vi "Write Target-FIFO 1ch.vi"(1 "FIFO In":refnum<k21>="FIFO-000", 5 "16IQ in":cluster{"I":fxp<+/-,18,1>, "Q":fxp<+/-,18,1>}[](array[cluster])=[{"I"=0.0, "Q"=0.0}, {"I"=0.0, "Q"=0.0}, {"I"=0.0, "Q"=0.0}, {"I"=0.0, "Q"=0.0}, {"I"=0.0, "Q"=0.0}, {"I"=0.0, "Q"=0.0}, {"I"=0.0, "Q"=0.0}, {"I"=0.0, "Q"=0.0}, {"I"=0.0, "Q"=0.0}, {"I"=0.0, "Q"=0.0}, {"I"=0.0, "Q"=0.0}, {"I"=0.0, "Q"=0.0}, {"I"=0.0, "Q"=0.0}, {"I"=0.0, "Q"=0.0}, {"I"=0.0, "Q"=0.0}, {"I"=0.0, "Q"=0.0}] {"I" format="%.18g"; "Q" format="%.18g"}, 9 "input valid":bool) -> (10 "Timed Out?":bool)   [LabVIEW 2015, in "DDC_7976R_v1.lvlib"]
uses:
  DDC_7976R_v1.lvlib
  <vilib>/rvi/Emulation/niFpgaSctlEmulationGetInTimedLoop.vi
  <vilib>/Utility/error.llb/Clear Errors.vi
  <vilib>/rvi/DataTransferAndStorage/Container/Common/niFpgaContainerExecOnDevCompGetState.vi
  <vilib>/rvi/Emulation/niFpgaEmulationIsFPGAContextNoSignature.vi
  <vilib>/rvi/errors/niFpgaSetErrorForExecOnDevCompSimple.vi
  <vilib>/rvi/eio/common/nirviEmuReportErrorAndStop.vi
  <vilib>/rvi/DataTransferAndStorage/Container/Common/niFpgaContainerGetUniqueNameForEmu.vi
  <vilib>/rvi/FIFO/Fifo_Resource/nirvififoEmulationSetSize.vi
  <vilib>/rvi/FIFO/Fifo_Resource/nirviFifoEmulationQueueMgr.vi
  <instcachedir>/0/nirviFifoEmulationQueueMgr_E5CAEC123FF24DC58D834DCA3CDAA9B5.lvgen/nirviFifoEmulationQueueMgr_E5CAEC123FF24DC58D834DCA3CDAA9B5_040.vi
  <vilib>/rvi/FIFO/Fifo_Resource/nirvififoEmulationDetermineInputValidOut.vi
  <vilib>/rvi/FIFO/Fifo_Resource/nirvififoEmulationCreateLock.vi
  <vilib>/rvi/Emulation/niFpgaProcessEmulError.vi
  <vilib>/rvi/FIFO/Fifo_Resource/nirvififoEmulationObtainLock.vi
  <vilib>/rvi/FIFO/Fifo_Resource/nirvififoEmulationReleaseLock.vi
  <vilib>/rvi/occurrence/nirviWaitOnOccurrenceBase.vi
  <vilib>/rvi/errors/nirviReportUnexpectedCaseInternalError.vi
  <vilib>/rvi/errors/nirviReportUnexpectedCaseInternalError (U32).vi
  <vilib>/rvi/interface/RandomDataEmulation/niFpgaRandomDataHandleErrors.vi
  <vilib>/rvi/DataTransferAndStorage/Container/XNode/niFpgaContainer.xnode
  <vilib>/rvi/FIFO/Fifo_Resource/niFpgaFifoEmulationRefIn.vi
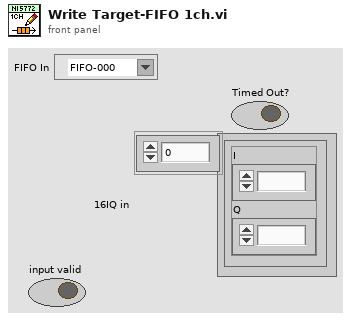
[diagram p1: front panel]
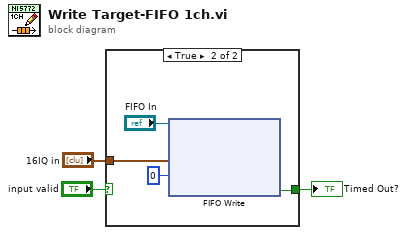
[diagram p0: block diagram]
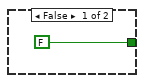
[diagram p2: hidden frame]
diagram:
  n1 = case shown="True" "input valid" {
    tunnel: [FALSE ("Timed Out?") w6] -> w2
    tunnel: "16IQ in" -> [_ w5]
    frame False {
    }
    frame True {
      n2 = xnode "FIFO Write"("Element"=w5, "Timeout"=0, "FIFO In"="FIFO In") -> ("Timed Out?"=w6:bool)  [unwired: 1 out]
    }
  }
  "Timed Out?" <- w2
